vi "determineParametersFilePath.vi"(8 "error in (no error)":errorcluster, 11 "Logger in":refnum<class "Log.lvclass">) -> (0 "error out":errorcluster, 3 "Logger out":refnum<class "Log.lvclass">)   [LabVIEW 2013, in "Log.lvclass"]
uses:
  Log.lvclass
  Log.lvclass/Log.ctl
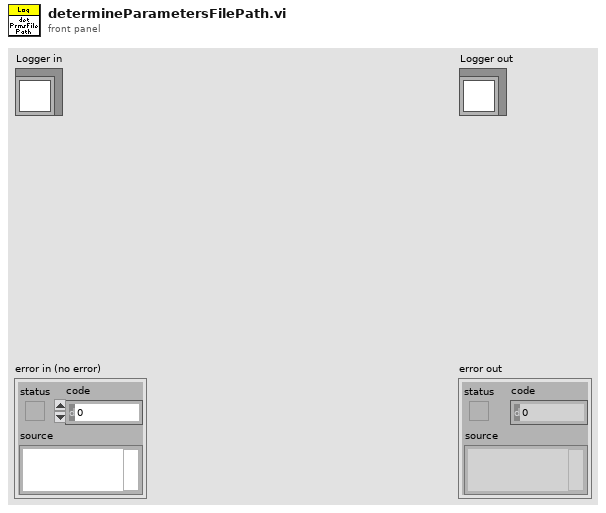
[diagram p1: front panel]
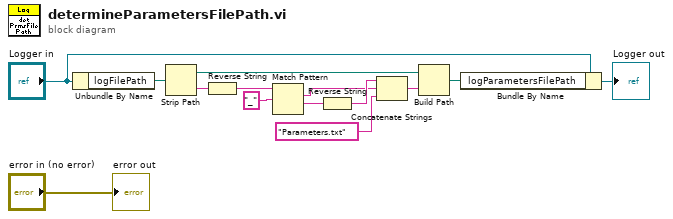
[diagram p0: block diagram]
diagram:
  n1 = Unbundle By Name("Logger in") -> ("logFilePath"=w1:path)
  n2 = Strip Path(path=w1) -> (stripped path=w7:path, name=w13:string)
  n3 = Reverse String(1:w13) -> (0:w12:string)
  n4 = Match Pattern(string=w12, regular expression="_") -> (match substring=w5:string, after substring=w6:string)  [unwired: 1 in, 2 out]
  n5 = Reverse String(1:w6) -> (0:w10:string)
  n6 = Concatenate Strings(w10, w5, "Parameters.txt" ("string")) -> (w8:string)
  n7 = Build Path(base path=w7, name or relative path=w8) -> (appended path=w3:path)
  n8 = Bundle By Name(cluster="Logger in", "logParametersFilePath"=w3) -> (→"Logger out":refnum<class "Log.lvclass">)
  "error out" <- "error in (no error)"
